vi "fgv_waypoint_curr_index.vi"(7 "cmd":enum16{"write", "read"}(ring), 11 "index in":i32) -> (3 "index out":i32)   [LabVIEW 2019]
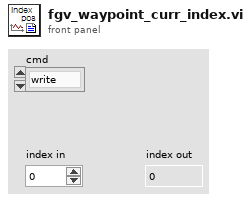
[diagram p1: front panel]
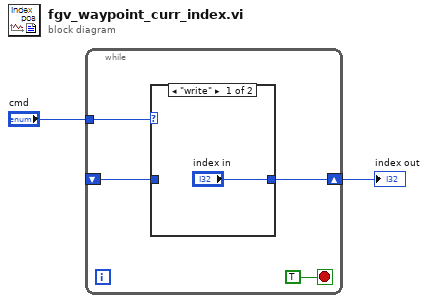
[diagram p0: block diagram]
diagram:
  n1 = while {
    tunnel: "cmd" -> [w5]
    shift-right: [w4] -> w1
    shift-left: _ -> [w3]
    stop <- TRUE stop-if-true
    n2 = case shown="\"write\"" w5 {
      tunnel: ["index in" w8] -> w4
      tunnel: w3 -> [_ w8]
      frame "write" {
      }
      frame "read", Default {
      }
    }
  }
  "index out" <- w1
